vi "Populate Objects Lists.vi"(8 "error in":errorcluster, 11 "UI Actor in":refnum<class "UI Actor.lvclass">) -> (0 "error out":errorcluster, 3 "UI Actor out":refnum<class "UI Actor.lvclass">)   [LabVIEW 2019, in "UI Actor.lvlib" / "UI Actor.lvclass"]
uses:
  UI Actor.lvclass
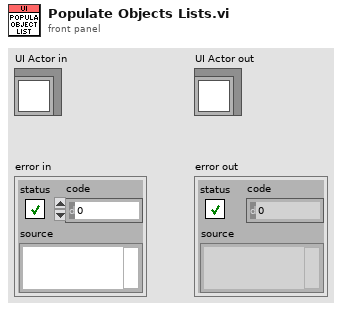
[diagram p1: front panel]
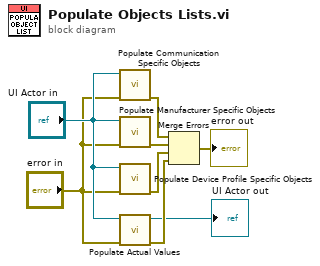
[diagram p0: block diagram]
diagram:
  n1 = call "Populate Communication Specific Objects.vi"("error in"="error in", "UI Actor in"="UI Actor in") -> ("error out"=w4:errorcluster)  [unwired: 9 in]
  n2 = call "Populate Manufacturer Specific Objects.vi"("error in"="error in", "UI Actor in"="UI Actor in") -> ("error out"=w3:errorcluster)  [unwired: 9 in]
  n3 = call "Populate Device Profile Specific Objects.vi"("error in"="error in", "UI Actor in"="UI Actor in") -> ("error out"=w2:errorcluster)  [unwired: 9 in]
  n4 = call-dynamic "Populate Actual Values.vi"("error in"="error in", "UI Actor in"="UI Actor in") -> ("error out"=w8:errorcluster, "UI Actor out"=→"UI Actor out":refnum<class "UI Actor.lvclass">)  [unwired: 8 in]
  n5 = Merge Errors(w4, w3, w2, w8) -> (→"error out":errorcluster)
